vi "Handle Supported Formats.vi"(8 "error in (no error)":errorcluster, 10 "FilePath":path, 11 "VI in":refnum<vi>) -> (0 "error out":errorcluster, 2 "dup FilePath":path, 3 "FileType Support Path":path)   [LabVIEW 2017, in "ImportExport.lvlib" / "ConfigFile.lvclass"]
uses:
  ConfigFile.lvclass
  <vilib>/Utility/error.llb/Error Cluster From Error Code.vi
  <vilib>/ErrorRing/Error Ring.xnode
  <vilib>/Utility/LVLibp/NI_PackedLibraryUtility.lvlib
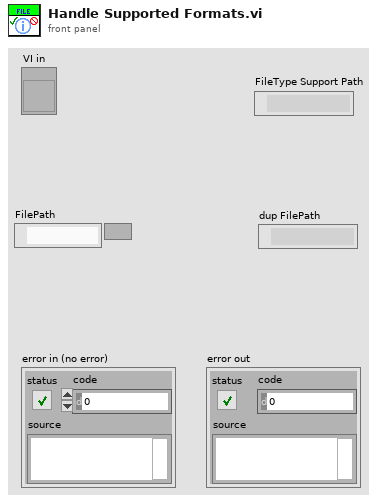
[diagram p1: front panel]
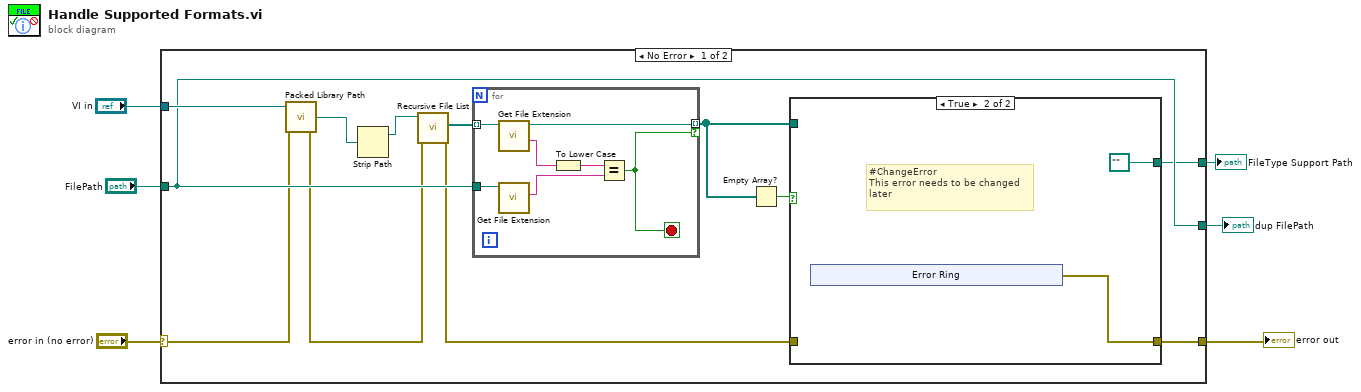
[diagram p0: block diagram]
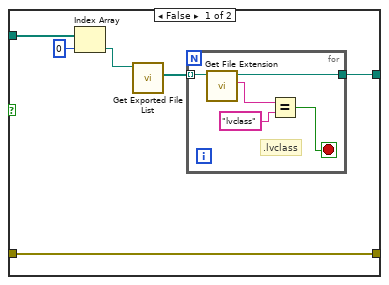
[diagram p2: hidden frame]
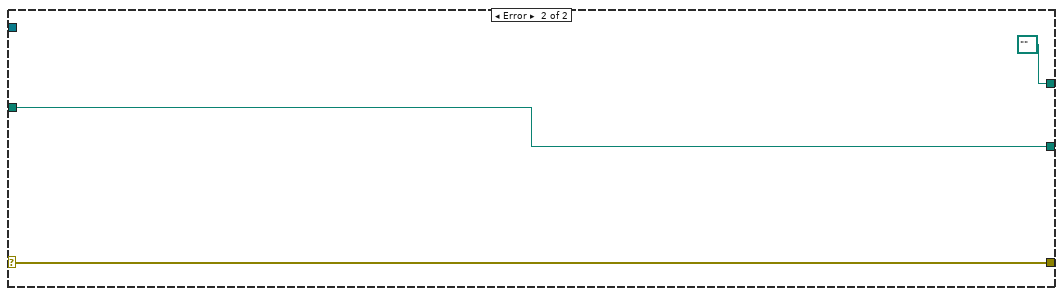
[diagram p3: hidden frame]
diagram:
  n1 = case shown="No Error" "error in (no error)" {
    selector: "error in (no error)" -> [w10 w45]
    tunnel: [w16 w45] -> w6
    tunnel: "VI in" -> [w17 _]
    tunnel: "FilePath" -> [w13 w44]
    tunnel: [w13 w44] -> w2
    tunnel: [w12 path "" ("dup file")] -> w1
    frame No Error {
      n2 = call <vilib>:"Packed Library Path.vi"("error in (no error)"=w10, "vi reference"=w17) -> ("error out"=w9:errorcluster, "packed library path"=w8:path)  [unwired: 1 in, 1 out]
      n3 = Strip Path(path=w8) -> (stripped path=w7:path)  [unwired: 1 out]
      n4 = call <vilib>:"Recursive File List.vi"("error in (no error)"=w9, "Folder Path"=w7) -> ("error out"=w11:errorcluster, "All Files in Dir"=w18:path[])  [unwired: 5 in, 3 out]
      n5 = for {
        tunnel: w18 -> [w42] mode=indexing
        tunnel: w13 -> [w38]
        tunnel: [w37] -> w14 mode=indexing if=w36
        stop <- w36 stop-if-true
        n6 = call <vilib>:"Get File Extension.vi"("file"=w42) -> ("filename without extension"=w39:string, "dup file"=w37:path)  [unwired: 6 in, 3 out]
        n7 = call <vilib>:"Get File Extension.vi"("file"=w38) -> ("lowercase file extension"=w41:string)  [unwired: 6 in, 4 out]
        n8 = To Lower Case(string=w39) -> (all lower case string=w40:string)
        n9 = Equal?(x=w40, y=w41) -> (x = y?=w36:bool)
      }
      n10 = Empty Array?(array=w14) -> (empty?=w15:bool)
      n11 = case shown="True" w15 {
        tunnel: w11 -> [w24 _]
        tunnel: [w24 w31] -> w16
        tunnel: w14 -> [w23 _]
        tunnel: [w19 path "" ("dup file")] -> w12
        frame False {
          n12 = Index Array(array=w23, index=0) -> (element=w21:path)
          n13 = call <vilib>:"Get Exported File List.vi"("packed library path"=w21) -> ("paths"=w20:path[])  [unwired: 8 in, 2 out]
          n14 = for {
            tunnel: w20 -> [w29] mode=indexing
            tunnel: [w25] -> w19
            stop <- w26 stop-if-true
            # ".lvclass"
            n15 = call <vilib>:"Get File Extension.vi"("file"=w29) -> ("lowercase file extension"=w27:string, "dup file"=w25:path)  [unwired: 6 in, 3 out]
            n16 = Equal?(x=w27, y="lvclass" ("lowercase file extension")) -> (x = y?=w26:bool)
          }
        }
        frame True {
          # "#ChangeError\nThis error needs to be changed\nlater"
          n17 = xnode "Error Ring"() -> ("error out"=w31:errorcluster)
        }
      }
    }
    frame Error {
    }
  }
  "error out" <- w6
  "dup FilePath" <- w2
  "FileType Support Path" <- w1
